vi "RGB To XYZ.vi"(3 "Blue":dbl, 4 "Green":dbl, 5 "Red":dbl) -> (0 "Z":dbl, 1 "Y":dbl, 2 "X":dbl)   [LabVIEW 2012]
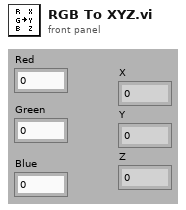
[diagram p1: front panel]
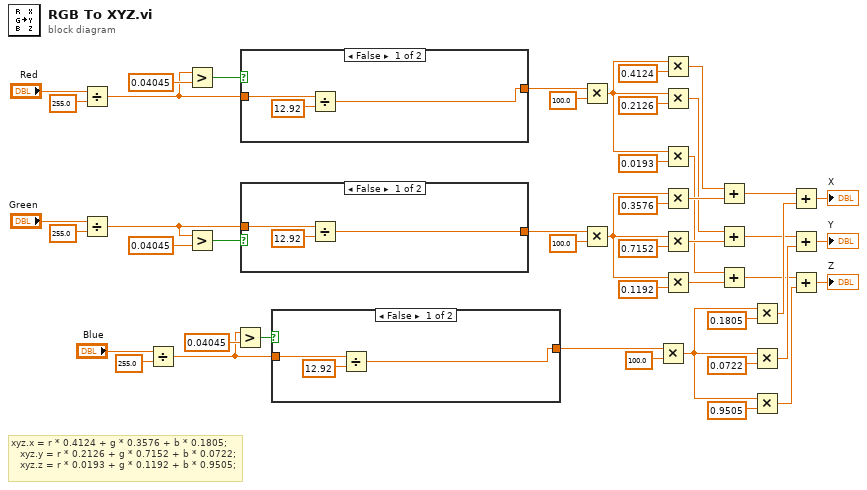
[diagram p0: block diagram]
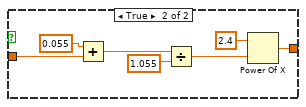
[diagram p2: hidden frame]
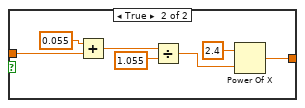
[diagram p3: hidden frame]
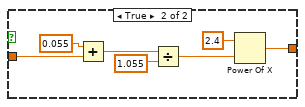
[diagram p4: hidden frame]
diagram:
  # "xyz.x = r * 0.4124 + g * 0.3576 + b * 0.1805;\n\t\t\txyz.y = r * 0.2126 + g * 0.7152 + b * 0.0722;\n\t\t\txyz.z = r * 0.0193 + g * 0.1192 + b * 0.9505;"
  n1 = Divide(x="Red", y=255.0) -> (x/y=w42:dbl)
  n2 = Divide(x="Green", y=255.0) -> (x/y=w35:dbl)
  n3 = Divide(x="Blue", y=255.0) -> (x/y=w34:dbl)
  n4 = Greater?(x=w42, y=0.04045) -> (0:w43:bool)
  n5 = Greater?(x=w35, y=0.04045) -> (0:w38:bool)
  n6 = Greater?(x=w34, y=0.04045) -> (0:w37:bool)
  n7 = case shown="False" w43 {
    tunnel: w42 -> [w51 w58]
    tunnel: [w49 w52] -> w33
    frame False {
      n8 = Divide(x=w51, y=12.92) -> (x/y=w49:dbl)
    }
    frame True {
      n9 = Add(x=0.055, y=w58) -> (x+y=w56:dbl)
      n10 = Divide(x=w56, y=1.055) -> (x/y=w54:dbl)
      n11 = Power Of X(1:w54, 2:2.4 ("y")) -> (0:w52:dbl)
    }
  }
  n12 = case shown="False" w38 {
    tunnel: [w60 w63] -> w29
    tunnel: w35 -> [w59 w62]
    frame False {
      n13 = Divide(x=w59, y=12.92) -> (x/y=w60:dbl)
    }
    frame True {
      n14 = Add(x=0.055, y=w62) -> (x+y=w67:dbl)
      n15 = Divide(x=w67, y=1.055) -> (x/y=w65:dbl)
      n16 = Power Of X(1:w65, 2:2.4 ("y")) -> (0:w63:dbl)
    }
  }
  n17 = case shown="False" w37 {
    tunnel: [w70 w73] -> w28
    tunnel: w34 -> [w69 w72]
    frame False {
      n18 = Divide(x=w69, y=12.92) -> (x/y=w70:dbl)
    }
    frame True {
      n19 = Add(x=0.055, y=w72) -> (x+y=w77:dbl)
      n20 = Divide(x=w77, y=1.055) -> (x/y=w75:dbl)
      n21 = Power Of X(1:w75, 2:2.4 ("y")) -> (0:w73:dbl)
    }
  }
  n22 = Multiply(x=w33, y=100.0) -> (x*y=w5:dbl)
  n23 = Multiply(x=w29, y=100.0) -> (x*y=w4:dbl)
  n24 = Multiply(x=w28, y=100.0) -> (x*y=w3:dbl)
  n25 = Multiply(x=w5, y=0.4124) -> (x*y=w24:dbl)
  n26 = Multiply(x=w5, y=0.2126) -> (x*y=w16:dbl)
  n27 = Multiply(x=w5, y=0.0193) -> (x*y=w9:dbl)
  n28 = Multiply(x=w4, y=0.3576) -> (x*y=w23:dbl)
  n29 = Multiply(x=w4, y=0.7152) -> (x*y=w17:dbl)
  n30 = Multiply(x=w4, y=0.1192) -> (x*y=w8:dbl)
  n31 = Add(x=w24, y=w23) -> (x+y=w22:dbl)
  n32 = Add(x=w16, y=w17) -> (x+y=w18:dbl)
  n33 = Add(x=w9, y=w8) -> (x+y=w7:dbl)
  n34 = Multiply(x=w3, y=0.1805) -> (x*y=w21:dbl)
  n35 = Multiply(x=w3, y=0.0722) -> (x*y=w19:dbl)
  n36 = Multiply(x=w3, y=0.9505) -> (x*y=w6:dbl)
  n37 = Add(x=w22, y=w21) -> (x+y=→"X":dbl)
  n38 = Add(x=w18, y=w19) -> (x+y=→"Y":dbl)
  n39 = Add(x=w7, y=w6) -> (x+y=→"Z":dbl)
